vi "CreateProcess (SubVI).vi"(8 "error in":errorcluster, 11 "AppContext in":T1={"VIRefToProcessTemplate"=refnum, "VIRefToThisVI"=refnum, "ProcessesList"=[], "VIRefToEnumProcess"=refnum, "VIRefTogetProcessViPath"=refnum, "ProcessManagement"={"EnumProcessState"=enum."Create process", "ProcessName"="", "PathToProcess"=path ""}, "VIRefToSetup"=refnum, "VIRefToStartProcess"=refnum, "ProcessConfig"={"File Path Control"=path "", "Timeout"=0.0, "viInitString"="", "State"=enum."Closed"}}) -> (0 "error out":errorcluster, 3 "AppContext out":T1={"VIRefToProcessTemplate"=refnum, "VIRefToThisVI"=refnum, "ProcessesList"=[], "VIRefToEnumProcess"=refnum, "VIRefTogetProcessViPath"=refnum, "ProcessManagement"={"EnumProcessState"=enum."Create process", "ProcessName"="", "PathToProcess"=path ""}, "VIRefToSetup"=refnum, "VIRefToStartProcess"=refnum, "ProcessConfig"={"File Path Control"=path "", "Timeout"=0.0, "viInitString"="", "State"=enum."Closed"}})   [LabVIEW 2011]
uses:
  Ctl/AppContext.ctl
  Ctl/EnumProcessState.ctl
  050 - CONFIG/20 - ExternalProcesses/paramsExternalProcesses.ctl
  Ctl/EnumThreePosition.ctl
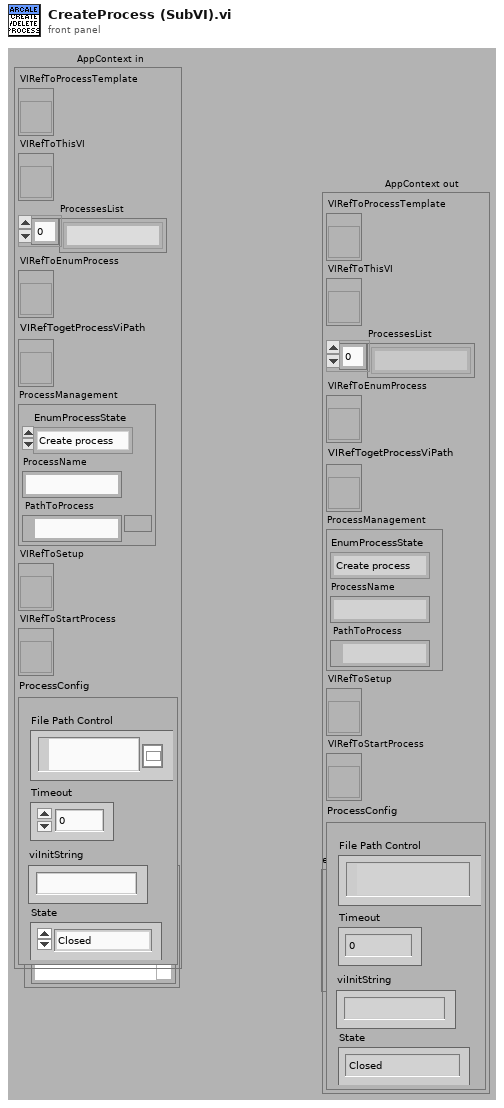
[diagram p1: front panel]
types:
  T1 = typedef "AppContext.ctl" = cluster{"VIRefToProcessTemplate":refnum<vi>, "VIRefToThisVI":refnum<vi>, "ProcessesList":string[], "VIRefToEnumProcess":refnum<vi>, "VIRefTogetProcessViPath":refnum<vi>, "ProcessManagement":cluster{"EnumProcessState":T2, "ProcessName":string, "PathToProcess":path}, "VIRefToSetup":refnum<vi>, "VIRefToStartProcess":refnum<vi>, "ProcessConfig":T3}
  T2 = typedef "EnumProcessState.ctl" = enum16{"Create process", "Delete process"}
  T3 = typedef "paramsExternalProcesses.ctl" = cluster{"File Path Control":path, "Timeout":dbl, "viInitString":string, "State":enum32{"Invalid", "Standard", "Closed", "Hidden", "Minimized", "Maximized"}}
  T4 = typedef "EnumThreePosition.ctl" = enum16{"DIVERS", "MAIN", "SPLASH SCREEN", "HMI", "EVENTS", "SCREENS", "CONFIG", "TOOLS", "ERRORS", "PROCESS"}
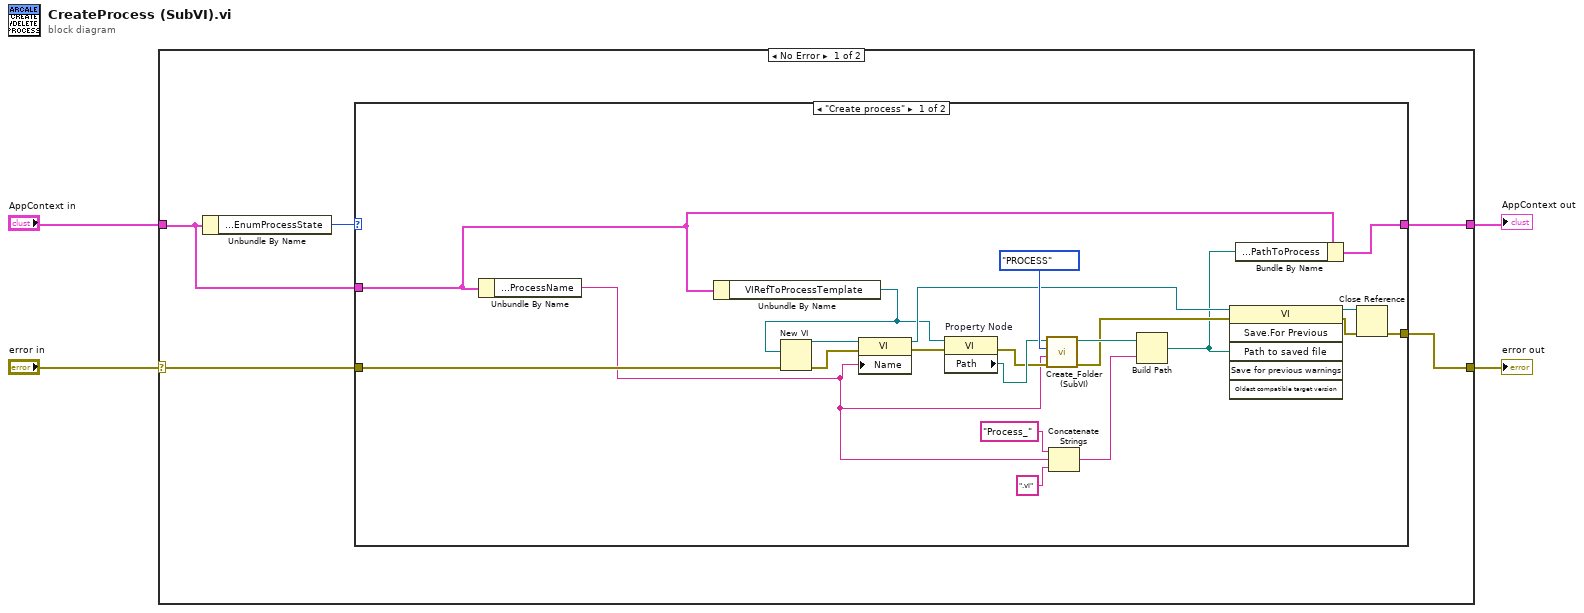
[diagram p0: block diagram]
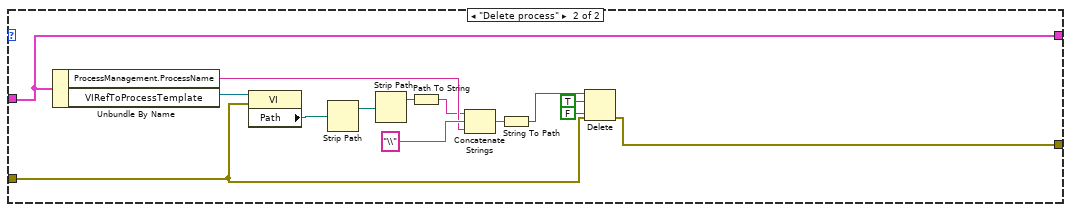
[diagram p2: hidden frame]
diagram:
  n1 = case shown="No Error" "error in" {
    selector: "error in" -> [w7 w45]
    tunnel: [w9 w45] -> w4
    tunnel: "AppContext in" -> [w5 w46]
    tunnel: [w8 w46] -> w2
    frame No Error {
      n2 = Unbundle By Name(w5) -> ("ProcessManagement.EnumProcessState"=w6:T2)
      n3 = case shown="\"Create process\"" w6 {
        tunnel: [w30 w42] -> w9
        tunnel: [w29 w37] -> w8
        tunnel: w7 -> [w12 w40]
        tunnel: w5 -> [w11 w37]
        frame "Create process" {
          n4 = Unbundle By Name(w11) -> ("ProcessManagement.ProcessName"=w10:string)
          n5 = Unbundle By Name(w11) -> ("VIRefToProcessTemplate"=w14:refnum<vi>)
          n6 = New VI(8:w12, 10:w14) -> (0:w27:errorcluster, 3:w28:refnum<vi>)  [unwired: 5 in]
          n7 = property class="VI"(reference=w28, error in=w27, "Name"=w10) -> (reference out=w15:refnum<vi>, error out=w26:errorcluster)
          n8 = property on="Property Node" class="VI"(reference=w14, error in=w26) -> (error out=w23:errorcluster, "Path"=w24:path)  [unwired: 1 out]
          n9 = call "Create_Folder (SubVI).vi"("error in"=w23, "Name"=w10, "Three position"=EnumThreePosition."PROCESS", "Path"=w24) -> ("error out"=w18:errorcluster, "created path"=w22:path)  [unwired: 6 in]
          n10 = Concatenate Strings("Process_" ("string"), w10, ".vi" ("string")) -> (w19:string)
          n11 = Build Path(base path=w22, name or relative path=w19) -> (appended path=w13:path)
          n12 = invoke class="VI" method="Save.For Previous"(reference=w15, error in=w18, "Path to saved file"=w13) -> (reference out=w17:refnum<vi>, error out=w16:errorcluster)  [unwired: 3 in, 4 out]
          n13 = Bundle By Name(cluster=w11, "ProcessManagement.PathToProcess"=w13) -> (w29:T1)
          n14 = Close Reference(reference=w17, error in (no error)=w16) -> (error out=w30:errorcluster)
        }
        frame "Delete process" {
          n15 = Unbundle By Name(w37) -> ("ProcessManagement.ProcessName"=w35:string, "VIRefToProcessTemplate"=w41:refnum<vi>)
          n16 = property class="VI"(reference=w41, error in=w40) -> ("Path"=w39:path)  [unwired: 2 out]
          n17 = Strip Path(path=w39) -> (stripped path=w38:path)  [unwired: 1 out]
          n18 = Strip Path(path=w38) -> (stripped path=w34:path)  [unwired: 1 out]
          n19 = Path To String(path=w34) -> (string=w33:string)
          n20 = Concatenate Strings(w33, "\\" ("string"), w35) -> (w32:string)
          n21 = String To Path(string=w32) -> (path=w31:path)
          n22 = Delete(path (use dialog)=w31, entire hierarchy (F)=TRUE, confirm (F)=FALSE, error in=w40) -> (error out=w42:errorcluster)  [unwired: 1 in, 2 out]
        }
      }
    }
    frame Error {
    }
  }
  "error out" <- w4
  "AppContext out" <- w2
